vi "Write WCM_limits.vi"(8 "error in (no error)":errorcluster, 10 "WCM_limits":T1, 11 "Experiment in":refnum<class "Experiment.lvclass">) -> (0 "error out":errorcluster, 3 "Experiment out":refnum<class "Experiment.lvclass">)   [LabVIEW 2015, in "Experiment.lvclass"]
uses:
  Experiment.lvclass
  dependecies/ControlsVIs/Clusters-def/Def_WCM_limits.ctl
  Experiment.lvclass/Experiment.ctl
  Oscilloscope/Oscilloscope.lvclass
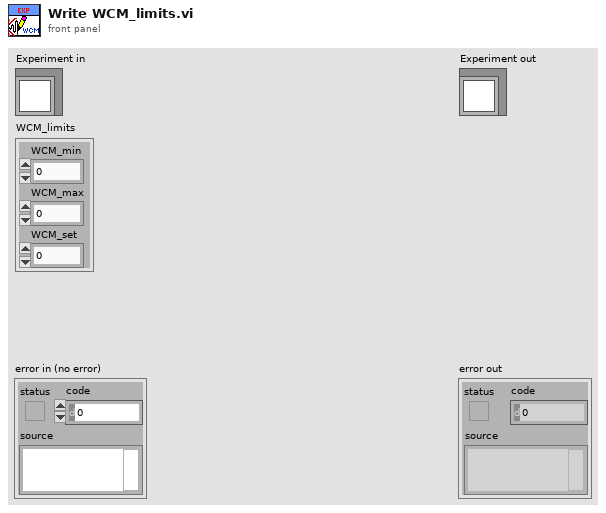
[diagram p1: front panel]
types:
  T1 = typedef "Oscilloscope.lvclass/Def_WCM_limits.ctl" = cluster{"WCM_min":dbl, "WCM_max":dbl, "WCM_set":dbl}
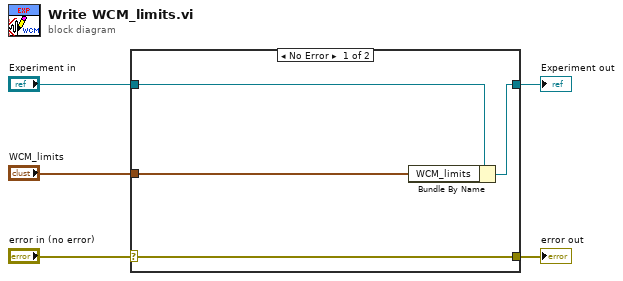
[diagram p0: block diagram]
diagram:
  n1 = case shown="No Error" "error in (no error)" {
    selector: "error in (no error)" -> [w9 w10]
    tunnel: [w9 w10] -> w4
    tunnel: [w7 w11] -> w2
    tunnel: "Experiment in" -> [w8 w11]
    tunnel: "WCM_limits" -> [w6 _]
    frame No Error {
      n2 = Bundle By Name(cluster=w8, "WCM_limits"=w6) -> (w7:refnum<class "Experiment.lvclass">)
    }
    frame Error {
    }
  }
  "error out" <- w4
  "Experiment out" <- w2
